vi "dht11_VisaSerial.vi"() -> ()   [LabVIEW 2018]
uses:
  <vilib>/Instr/_visa.llb/VISA Configure Serial Port (Instr).vi
panel:
  in  "Tab Control":enum32{"Page 1", "TEMPERATURA", "HUMEDAD"}(tab)
  in  "VISA resource name":refnum<visa-resource-name>
  in  "baud rate (115200)":u32=9600
  out "TEMPERATURA C":dbl(slide) scale=0.0..100.0
  out "HUMEDAD":dbl(slide) scale=0.0..100.0
  in  "REFERENCIA T":dbl(slide) scale=0.0..100.0
  out "GRAFICA TEMP":dynamicdata(graph)
  in  "stop":bool
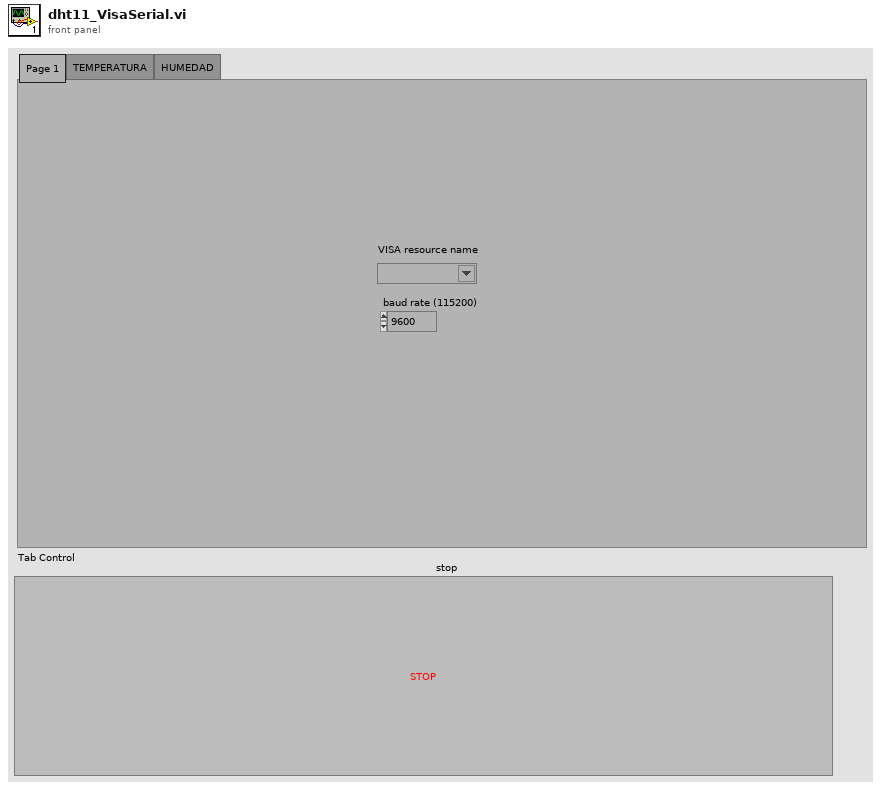
[diagram p1: front panel]
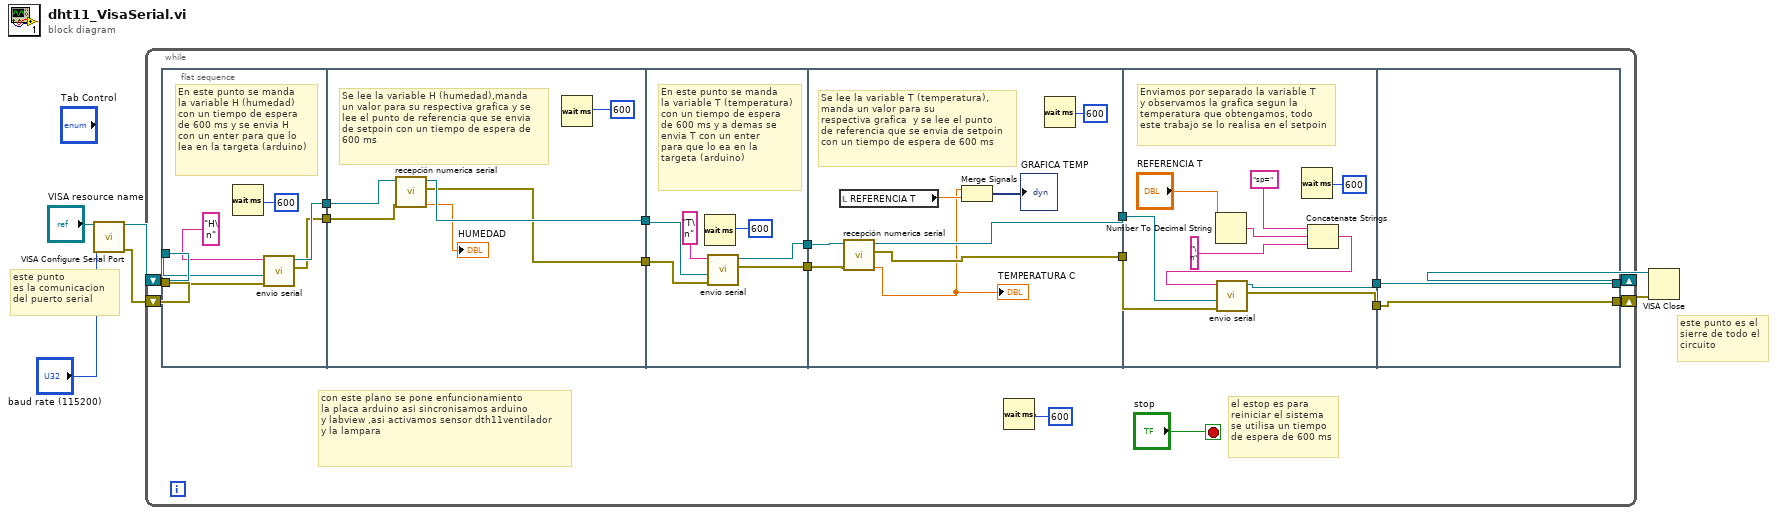
[diagram p0: block diagram]
diagram:
  # "este punto es el\nsierre de todo el \ncircuito"
  # "este punto\nes la comunicacion \ndel puerto serial"
  n1 = call-poly "VISA Configure Serial Port"("VISA resource name"="VISA resource name", "baud rate (9600)"="baud rate (115200)") -> ("VISA resource name out"=w4:refnum<visa-resource-name>, "error out"=w5:errorcluster)  [unwired: 12 in]
  n2 = while {
    shift-right: [w7] -> w2
    shift-left: w5 -> [w18]
    shift-right: [w8] -> w3
    shift-left: w4 -> [w22]
    stop <- "stop" stop-if-true
    # "con este plano se pone enfuncionamiento\nla placa arduino asi sincronisamos arduino \ny labview ,asi activamos sensor dth11ventilador\ny la lampara"
    # "el estop es para\nreiniciar el sistema\nse utilisa un tiempo\nde espera de 600 ms"
    n3 = flat-sequence {
      tunnel: w18 -> [w23]
      tunnel: w22 -> [w24]
      tunnel: [w26] -> w20
      tunnel: [w25] -> w19
      tunnel: w20 -> [w33]
      tunnel: w19 -> [w34]
      tunnel: [w32] -> w17
      tunnel: [w31] -> w16
      tunnel: w17 -> [w40]
      tunnel: w16 -> [w39]
      tunnel: [w36] -> w15
      tunnel: [w35] -> w14
      tunnel: w15 -> [w48]
      tunnel: w14 -> [w47]
      tunnel: [w46] -> w12
      tunnel: [w45] -> w11
      tunnel: w12 -> [w58]
      tunnel: w11 -> [w49]
      tunnel: [w52] -> w10
      tunnel: [w51] -> w9
      tunnel: w10 -> [w60]
      tunnel: w9 -> [w59]
      tunnel: [w60] -> w8
      tunnel: [w59] -> w7
      frame #0 {
        # "En este punto se manda\nla variable H (humedad)\ncon un tiempo de espera \nde 600 ms y se envia H \ncon un enter para que lo \nlea en la targeta (arduino)"
        n4 = Wait (ms)(milliseconds to wait=u32 600) -> ()  [unwired: 1 out]
        n5 = call "envio serial.vi"("error"=w23, "VISA resource name"=w24, "Arduino Envio"="H\n") -> ("error out"=w25:errorcluster, "VISA resource name out"=w26:refnum<visa-resource-name>)  [unwired: 3 in]
      }
      frame #1 {
        # "Se lee la variable H (humedad),manda\nun valor para su respectiva grafica y se\nlee el punto de referencia que se envia \nde setpoin con un tiempo de espera de\n600 ms"
        n6 = call "recepción numerica serial.vi"("error out"=w34, "VISA resource name out"=w33) -> ("number"=→"HUMEDAD":dbl, "error out 2"=w31:errorcluster, "VISA resource name out 2"=w32:refnum<visa-resource-name>)  [unwired: 2 in, 1 out]
        n7 = Wait (ms)(milliseconds to wait=u32 600) -> ()  [unwired: 1 out]
      }
      frame #2 {
        # "En este punto se manda\nla variable T (temperatura)\ncon un tiempo de espera \nde 600 ms y a demas se \nenvia T con un enter\npara que lo ea en la \ntargeta (arduino)"
        n8 = Wait (ms)(milliseconds to wait=u32 600) -> ()  [unwired: 1 out]
        n9 = call "envio serial.vi"("error"=w39, "VISA resource name"=w40, "Arduino Envio"="T\n") -> ("error out"=w35:errorcluster, "VISA resource name out"=w36:refnum<visa-resource-name>)  [unwired: 3 in]
      }
      frame #3 {
        # "Se lee la variable T (temperatura),\nmanda un valor para su \nrespectiva grafica  y se lee el punto\nde referencia que se envia de setpoin\ncon un tiempo de espera de 600 ms"
        n10 = local read "REFERENCIA T"() -> (w42:dbl)
        n11 = call "recepción numerica serial.vi"("error out"=w47, "VISA resource name out"=w48) -> ("number"=w41:dbl, "error out 2"=w45:errorcluster, "VISA resource name out 2"=w46:refnum<visa-resource-name>)  [unwired: 2 in, 1 out]
        "TEMPERATURA C" <- w41
        n12 = Merge Signals(w41, w42) -> (→"GRAFICA TEMP":dynamicdata)
        n13 = Wait (ms)(milliseconds to wait=u32 600) -> ()  [unwired: 1 out]
      }
      frame #4 {
        # "Enviamos por separado la variable T\ny observamos la grafica segun la \ntemperatura que obtengamos, todo \neste trabajo se lo realisa en el setpoin"
        n14 = Number To Decimal String(number="REFERENCIA T") -> (decimal integer string=w54:string)  [unwired: 1 in]
        n15 = Wait (ms)(milliseconds to wait=u32 600) -> ()  [unwired: 1 out]
        n16 = Concatenate Strings("sp=" ("string"), w54, "\n" ("string")) -> (w57:string)
        n17 = call "envio serial.vi"("error"=w49, "VISA resource name"=w58, "Arduino Envio"=w57) -> ("error out"=w51:errorcluster, "VISA resource name out"=w52:refnum<visa-resource-name>)  [unwired: 3 in]
      }
      frame #5 {
      }
    }
    n18 = Wait (ms)(milliseconds to wait=u32 600) -> ()  [unwired: 1 out]
  }
  n19 = VISA Close(VISA resource name=w3, error in (no error)=w2) -> ()  [unwired: 1 out]
